vi "TrapezoidaSignal.vi"() -> ()   [LabVIEW 2017]
uses:
  <vilib>/imath/engines/lvmath2/RunTimeEngine/Managers/WorkSpace/UID Generator.vi
  <vilib>/imath/engines/lvmath2/RunTimeEngine/RunTimeType/NIMS_RunTimeType_From StrictType (excl LVString).vi
  <instcachedir>/0/NIMS_RunTimeType_From StrictType (excl LVString)_1019F277F0A747EDBCA0F6C52CA54500.lvgen/NIMS_RunTimeType_From StrictType (excl LVString)_1019F277F0A747EDBCA0F6C52CA54500_000.vi
  <vilib>/imath/engines/lvmath2/RunTimeEngine/LocalVariableDefStatement/MC_LocalVariableDefStatement_Display.vi
  <vilib>/imath/engines/lvmath2/RunTimeEngine/RangeToken/NIMS_Range.vi
  <instcachedir>/0/NIMS_Range_69CB9AAD882742A19CF7E739BE79952C.lvgen/NIMS_Range_69CB9AAD882742A19CF7E739BE79952C_000.vi
  <vilib>/imathl/engines/lvmath/Functions/Error Handling/Create Error.vi
  <vilib>/imath/engines/lvmath2/RunTimeEngine/Managers/SymbolTable/Clear UID.vi
  <vilib>/imath/engines/lvmath2/RunTimeEngine/NodeEndStatement/NIMS_NodeEndStatement_Output.vi
  <instcachedir>/0/NIMS_NodeEndStatement_Output_53EC0D466D134D7ABD903AC30B43404B.lvgen/NIMS_NodeEndStatement_Output_53EC0D466D134D7ABD903AC30B43404B_005.vi
  <vilib>/imath/engines/lvmath2/RunTimeEngine/ErrorHandling/NIMS_Finalize Error.vi
  <vilib>/imath/engines/lvmath2/RunTimeEngine/Managers/SymbolTable/NIMS_WorkSpace.lvlib
panel:
  out "size(s)":i32
  out "XY Graph":cluster{"t":dbl[], "y":dbl[]}(graph)
  in  "Signal Paremeters":T1={"Initial Ctr. Ratio"=0.1, "Maximum Ctr.Ratio"=0.2, "T1 - Period of RampUP"=10.0, "T2 - Period of Steady"=10.0, "T3 - Period of RampDown"=10.0}
  in  "Digitizing Parameters":T2
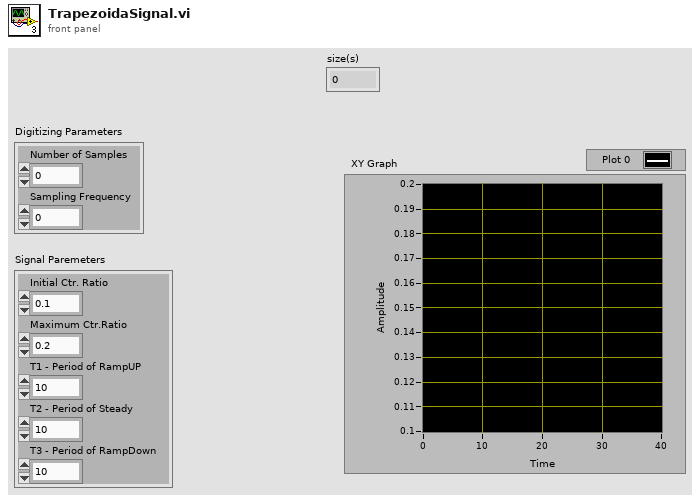
[diagram p1: front panel]
types:
  T1 = cluster{"Initial Ctr. Ratio":dbl, "Maximum Ctr.Ratio":dbl, "T1 - Period of RampUP":dbl, "T2 - Period of Steady":dbl, "T3 - Period of RampDown":dbl}
  T2 = cluster{"Number of Samples":dbl, "Sampling Frequency":dbl}
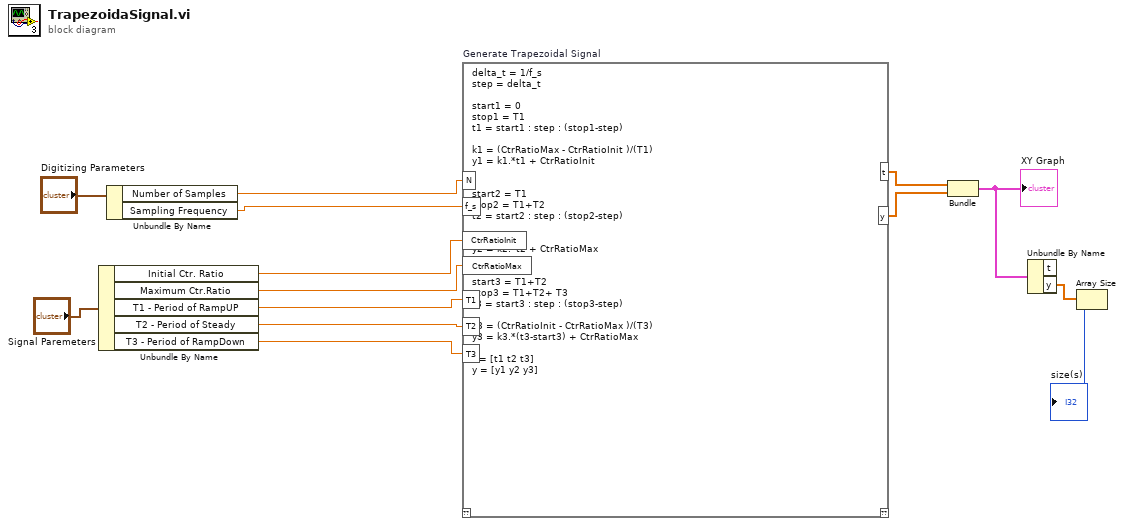
[diagram p0: block diagram]
diagram:
  n1 = Unbundle By Name("Signal Paremeters") -> ("Initial Ctr. Ratio"=w6:dbl, "Maximum Ctr.Ratio"=w10:dbl, "T1 - Period of RampUP"=w9:dbl, "T2 - Period of Steady"=w8:dbl, "T3 - Period of RampDown"=w7:dbl)
  n2 = Unbundle By Name("Digitizing Parameters") -> ("Number of Samples"=w13:dbl, "Sampling Frequency"=w12:dbl)
  n3 = mathscript code="delta_t = 1/f_s\nstep = delta_t\n\nstart1 = 0\nstop1 = T1\nt1 = start1 : step : (stop1-step)\n\nk1 = (CtrRatioMax - CtrRatioInit )/(T1)\ny1 = k1.*t1 + CtrRatioInit\n\n\nstart2 = T1\nstop2 = T1+T2\nt2 = start2 : step : (stop2-step)\n\nk2 = 0\ny2 = k2.*t2 + CtrRatioMax\n\n\nstart3 = T1+T2\nstop3 = T1+T2+ T3\nt3 = start3 : step : (stop3-step)\n\nk3 = (CtrRatioInit - CtrRatioMax )/(T3)\ny3 = k3.*(t3-start3) + CtrRatioMax\n\nt = [t1 t2 t3]\ny = [y1 y2 y3]" "Generate Trapezoidal Signal"("N"=w13, "f_s"=w12, "CtrRatioMax"=w10, "T1"=w9, "T2"=w8, "T3"=w7, "CtrRatioInit"=w6) -> ("t"=w5:dbl[], "y"=w4:dbl[])  [unwired: 1 in, 1 out]
  n4 = Bundle("t"=w5, "y"=w4) -> (w3:cluster{"t":dbl[], "y":dbl[]})  [unwired: 1 in]
  "XY Graph" <- w3
  n5 = Unbundle By Name(w3) -> ("y"=w2:dbl[])  [unwired: 1 out]
  n6 = Array Size(array=w2) -> (size(s)=→"size(s)":i32)
